vi "Define Columns.vi"(10 "Enum Array":refnum<vi>[](array[refnum])) -> (2 "Column Definition":T1[](array[typedef]) {"MinWidth" min=2 step=1; "AutoSizeMode" items=["None"=1, "ColumnHeader"=2, "AllCellsExceptHeader"=4, "AllCells"=6, "DisplayedCellsExceptHeader"=8, "DisplayedCells"=10, "Fill"=16]; "FillWeight" min=1 max=100})   [LabVIEW 2014, in "OPC UA Client editor node.lvclass"]
doc: "This VI defines the columns that will be used in the table. You can specify the column type and the dimensions if the columns."
uses:
  OPC UA Client editor node.lvclass
  <vilib>/NI/DCAF/Tag Editor Core/Table API/Column/Column Descriptor.ctl
  <vilib>/NI/DCAF/Tag Editor Core/Table API/Column/Column.lvclass
  <vilib>/NI/DCAF/Tag Editor Core/Table API/Column/Column Type.ctl
  <vilib>/NI/Tag Bus/tag/Data Type.ctl
  <vilib>/NI/DCAF/Tag Editor Core/Table API/Table Manager/Call Back Ref Type Def.ctl
  <vilib>/NI/DCAF/Tag Editor Core/Configuration Editor/Classes/Engine Parent/Engine Parent Editor Node.lvclass
  <vilib>/NI/DCAF/Tag Editor Core/Configuration Editor/Classes/Module editor node/module editor node.lvclass
  Callback Change Channel Name.vi
  Callback Change Direction.vi
  Callback Change Tag.vi
  Callback Change UA Data Type.vi
  <vilib>/NI/DCAF/Tag Editor Core/Table API/Mapping Column/Mapping Column.lvclass
  <vilib>/NI/DCAF/Tag Editor Core/Table API/String Column/String Column.lvclass
  <vilib>/NI/DCAF/Tag Editor Core/Table API/Listbox Enum Column/List Box Enum Column.lvclass
  <vilib>/NI/Tag Bus/tag/tag descriptor.lvclass
  <vilib>/NI/DCAF/Tag Editor Core/Table API/Table Manager/Table Manager.lvclass
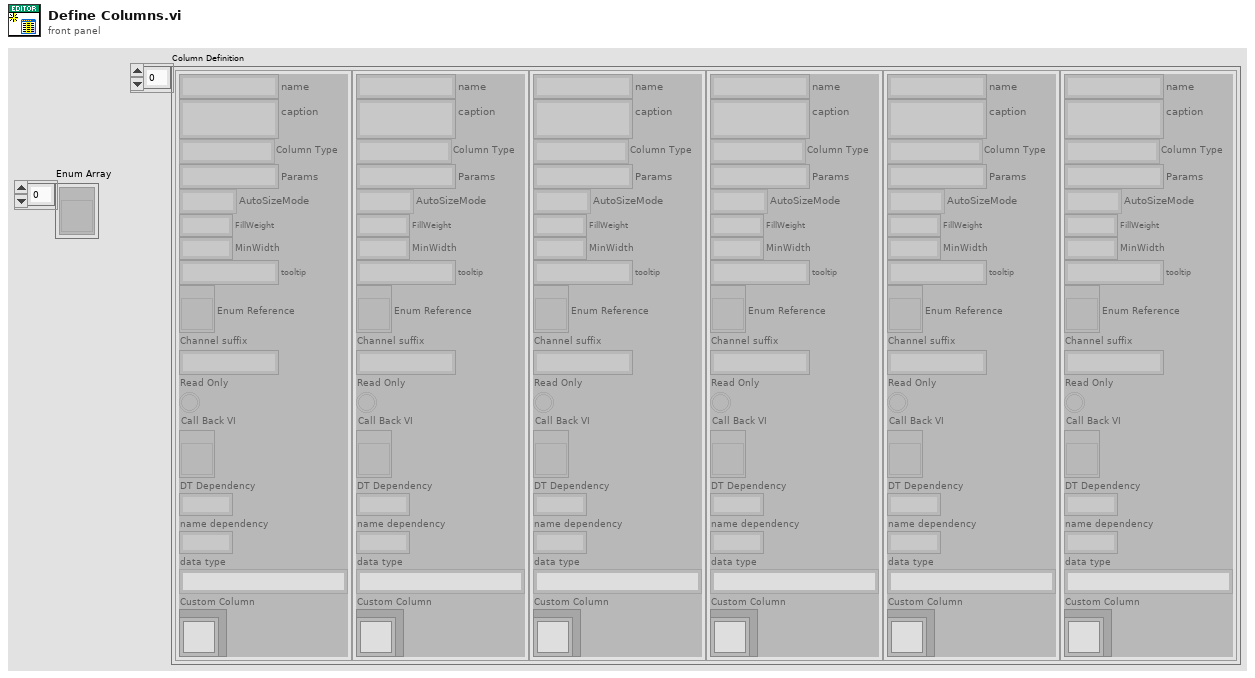
[diagram p1: front panel]
types:
  T1 = typedef "Table Manager.lvlib/Column.lvclass/Column Descriptor.ctl" = cluster{"name":string, "caption":string, "Column Type":T2, "Params":string, "AutoSizeMode":i32, "FillWeight":sgl, "MinWidth":u32, "tooltip":string, "Enum Reference":refnum<vi>, "Channel suffix":string, "Read Only":bool, "Call Back VI":T3, "DT Dependency":i32, "name dependency":i32, "data type":T4, "Custom Column":refnum<class "Column.lvclass">}
  T2 = typedef "Table Manager.lvlib/Column.lvclass/Column Type.ctl" = enum16{"String", "Mapping", "Enum", "Custom"}
  T3 = typedef "Table Manager.lvlib/Table Manager.lvclass/Call Back Ref Type Def.ctl" = refnum<vi>
  T4 = typedef "tag bus.lvlib/tag descriptor.lvclass/Data Type.ctl" = enum16{"Double", "Single", "I64", "I32", "I16", "I8", "U64", "U32", "U16", "U8", "Boolean", "String", "Array of Double", "Array of Single", "Array of I64", "Array of I32", "Array of I16", "Array of I8", "Array of U64", "Array of U32", "Array of U16", "Array of U8", "Array of Boolean", "Array of String"}
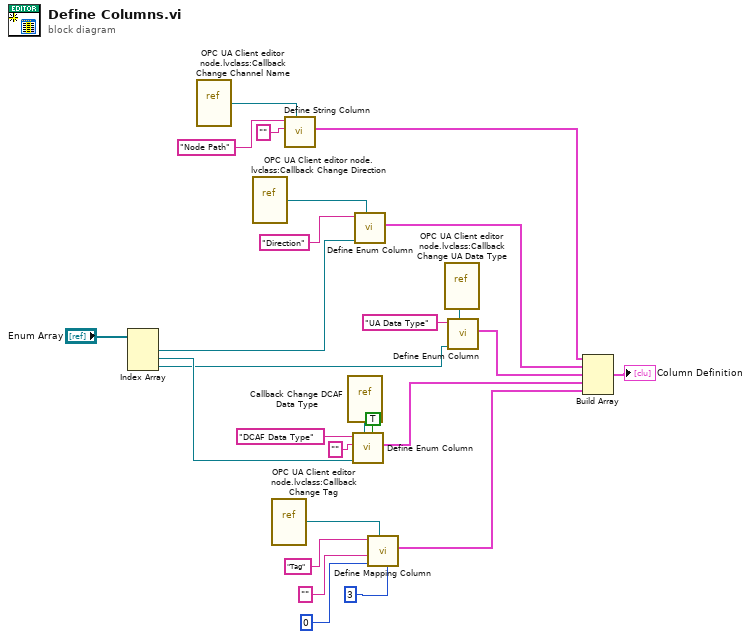
[diagram p0: block diagram]
diagram:
  n1 = Index Array(array="Enum Array") -> (element #1=w17:refnum<vi>, element #2=w14:refnum<vi>, element #3=w2:refnum<vi>)  [unwired: 3 in]
  n2 = vi-ref "OPC UA Client editor node.lvclass:Callback Change Channel Name.vi"() -> (w12:refnum<vi>)
  n3 = vi-ref "OPC UA Client editor node.lvclass:Callback Change Direction.vi"() -> (w11:refnum<vi>)
  n4 = vi-ref "OPC UA Client editor node.lvclass:Callback Change Tag.vi"() -> (w9:refnum<vi>)
  n5 = call <vilib>:"Define String Column.vi"("Call Back VI"=w12, "Caption"="", "Name"="Node Path" ("name")) -> ("Column Descriptor out"=w1:T1)  [unwired: 8 in]
  n6 = vi-ref "Callback Change DCAF Data Type.vi"() -> (w10:refnum<vi>)
  n7 = call <vilib>:"Define Enum Column.vi"("Read Only (F)"=TRUE, "Call Back VI"=w10, "Enum Reference"=w14, "Caption"="", "Name"="DCAF Data Type" ("name")) -> ("Column Descriptor out"=w6:T1)  [unwired: 6 in]
  n8 = call <vilib>:"Define Enum Column.vi"("Call Back VI"=w11, "Enum Reference"=w17, "Name"="Direction" ("name")) -> ("Column Descriptor out"=w13:T1)  [unwired: 8 in]
  n9 = call <vilib>:"Define Mapping Column.vi"("DT Dependency (-1)"=3 ("DT Dependency"), "Call Back VI"=w9, "name dependency"=0, "Channel suffix"="" ("string"), "name"="Tag") -> ("Column Descriptor out"=w7:T1)  [unwired: 6 in]
  n10 = vi-ref "OPC UA Client editor node.lvclass:Callback Change UA Data Type.vi"() -> (w4:refnum<vi>)
  n11 = call <vilib>:"Define Enum Column.vi"("Call Back VI"=w4, "Enum Reference"=w2, "Name"="UA Data Type" ("name")) -> ("Column Descriptor out"=w3:T1)  [unwired: 8 in]
  n12 = Build Array(w1, w13, w3, w6, w7) -> (→"Column Definition":T1[])
